vi "Scrip_execution.vi"   [LabVIEW 2024]
types:
  T1 = cluster{"元素":string, "元素 2":string, "元素 3":string, "元素 4":string, "元素 5":string, "元素 6":string, "元素 7":string, "元素 8":string, "元素 9":string, "元素 10":string, "元素 11":string, "元素 12":string, "元素 13":string, "元素 14":string, "元素 15":string}[]
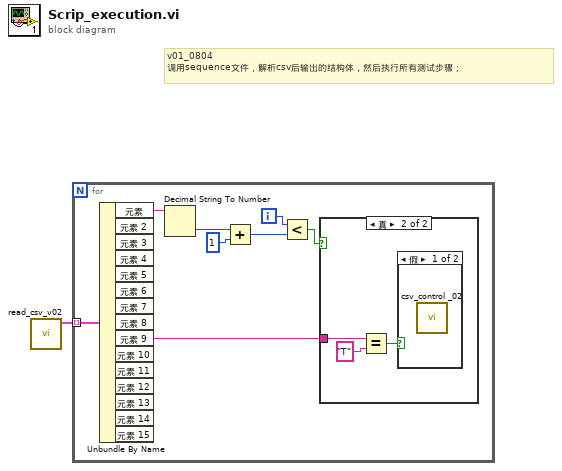
[diagram p0: block diagram]
diagram:
  # "v01_0804\n调用sequence文件，解析csv后输出的结构体，然后执行所有测试步骤；"
  n1 = call "read_csv_v02.vi"() -> ("目标结构体数组"=w1:T1)  [unwired: 11 in]
  n2 = for {
    tunnel: w1 -> [w9] mode=indexing
    i -> [w3]
    n3 = Unbundle By Name(w9) -> ("元素"=w7:string, "元素 9"=w8:string)  [unwired: 13 out]
    n4 = Decimal String To Number(string=w7) -> (number=w6:i32)  [unwired: 2 in, 1 out]
    n5 = Add(x=w6, y=1) -> (x+y=w2:i32)
    n6 = Less?(x=w3, y=w2) -> (x < y?=w5:bool)
    n7 = case shown="真" w5 {
      tunnel: w8 -> [_ w10]
      frame False {
      }
      frame True {
        n8 = Equal?(x=w10, y="T") -> (x = y?=w11:bool)
        n9 = case shown="假" w11 {
          frame False {
            n10 = call "csv_control _02.vi"() -> ()  [unwired: 11 in, 1 out]
          }
          frame True {
          }
        }
      }
    }
  }
